vi "alg_rank (SubVI).vi"(8 "에러 입력(에러 없음)":errorcluster, 11 "matrix":dbl[][](array[numeric])=[[1.0, 2.0], [3.0, 4.0]]) -> (0 "에러 출력":errorcluster, 2 "ans":i32, 3 "참조 번호 출력":refnum<k35>)   [LabVIEW 2018]
uses:
  PythonConfigGlobal.vi
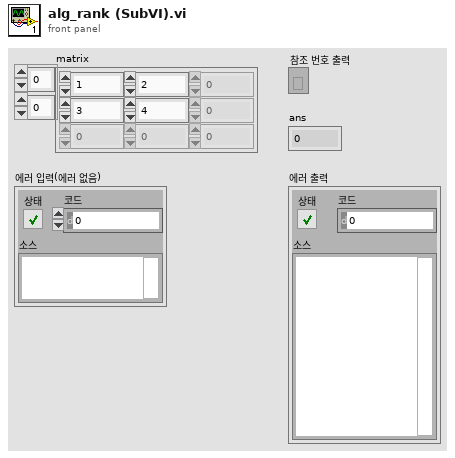
[diagram p1: front panel]
types:
  T1 = cluster{"session out":refnum<k35>, "appended path":path}
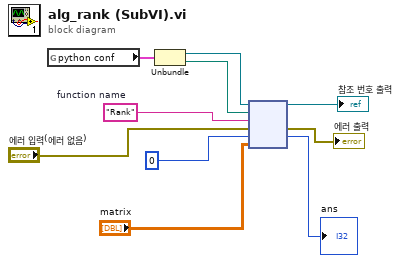
[diagram p0: block diagram]
diagram:
  w6 = "Rank"  # function name
  n1 = global read "PythonConfigGlobal.vi" "python conf"() -> (w3:T1)
  n2 = Unbundle(w3) -> ("session out"=w5:refnum<k35>, "appended path"=w4:path)
  n3 = node(w5, w4, w6, "에러 입력(에러 없음)", 0, "matrix") -> (→"참조 번호 출력":refnum<k35>, →"에러 출력":errorcluster, →"ans":i32)  [unwired: 1 in, 2 out]
